vi "Word_Insert_Panel.vi"(0 "Word.Document":refnum<k7>, 1 "Word.InlineShapes":refnum<k7>, 2 "visible area only":bool, 3 "Image depth":u16(ring)=3 items=["B&W", "4 bits", "8 bits", "24 bits"], 5 "VI name":string, 9 "alignment (default)":T1, 11 "Error in":errorcluster, 12 "Insertion point":u16(ring)=1 items=["begining of document", "end of document", "bookmark"], 13 "bookmark name":string, 14 "image file type(.jpg)":enum16{".jpg", ".png"}(ring)) -> (8 "Start out":i32, 10 "End out":i32, 15 "Error out":errorcluster)   [LabVIEW 2020, in "NI_ReportGenerationToolkit.lvlib"]
uses:
  <vilib>/addons/_office/NI_ReportGenerationToolkit.lvlib
  <vilib>/Utility/NIReport.llb/HTML Report Image Alignment.ctl
  <vilib>/Utility/NIReport.llb/NI_ReportGenerationCore.lvlib
panel:
  # "Image"
  # "Position"
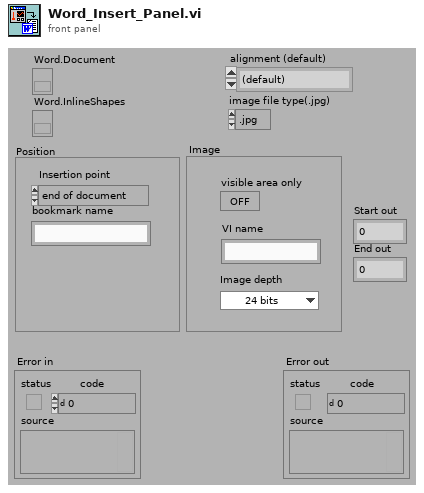
[diagram p1: front panel]
types:
  T1 = typedef "NI_ReportGenerationCore.lvlib/HTML Report Image Alignment.ctl" = enum16{"(default)", "LEFT", "RIGHT", "TOP", "TEXTTOP", "MIDDLE", "ABSMIDDLE", "BASELINE", "BOTTOM", "ABSBOTTOM"}
  T2 = typedef "imagedata.ctl" = cluster{"image type":i32, "image depth":i32, "image":u8[], "mask":u8[], "colors":u32[], "Rectangle":cluster{"left":i16, "top":i16, "right":i16, "bottom":i16}}
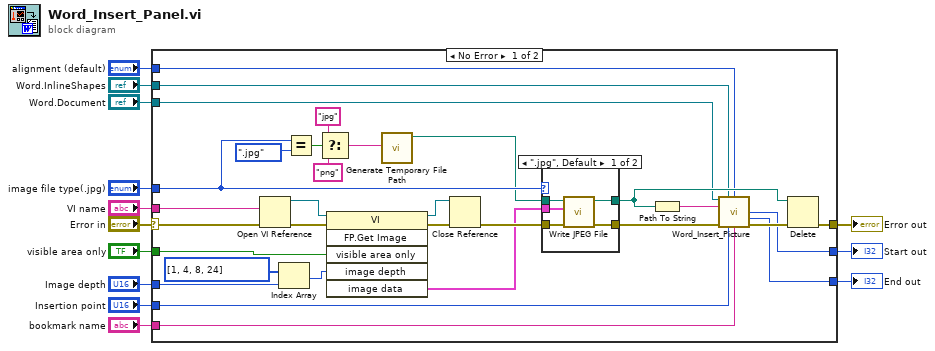
[diagram p0: block diagram]
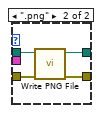
[diagram p2: hidden frame]
diagram:
  n1 = case shown="No Error" "Error in" {
    selector: "Error in" -> [w14 w54]
    tunnel: "VI name" -> [w44 _]
    tunnel: "Image depth" -> [w42 _]
    tunnel: [w41 w54] -> w11
    tunnel: "visible area only" -> [w37 _]
    tunnel: "Word.Document" -> [w35 _]
    tunnel: "Insertion point" -> [w33 _]
    tunnel: "bookmark name" -> [w32 _]
    tunnel: [w29 _] -> w6
    tunnel: [w28 _] -> w5
    tunnel: "alignment (default)" -> [w27 _]
    tunnel: "Word.InlineShapes" -> [w23 _]
    tunnel: "image file type(.jpg)" -> [w17 _]
    frame No Error {
      n2 = Open VI Reference(vi path=w44, error in (no error)=w14) -> (vi reference=w39:refnum<vi>, error out=w36:errorcluster)  [unwired: 4 out]
      n3 = Index Array(array=i32[] [1, 4, 8, 24] ("Array Constant"), index=w42) -> (element=w38:i32)
      n4 = Equal?(x=w17, y=enum16{".jpg", ".png"}.".jpg") -> (x = y?=w21:bool)
      n5 = Select(t="jpg", s=w21, f="png") -> (s? t:f=w20:string)
      n6 = invoke class="VI" method="FP.Get Image"(reference=w39, error in=w36, "visible area only"=w37, "image depth"=w38) -> (reference out=w24:refnum<vi>, error out=w26:errorcluster, "image data"=w15:T2)  [unwired: 2 in, 3 out]
      n7 = call <vilib>:"Generate Temporary File Path.vi"("Temporary File Extension (tmp)"=w20) -> ("Unique Temporary File Path"=w16:path)  [unwired: 1 in, 9 out]
      n8 = Close Reference(reference=w24, error in (no error)=w26) -> (error out=w25:errorcluster)
      n9 = case shown="\".jpg\", Default" w17 {
        tunnel: w16 -> [w47 w53]
        tunnel: w25 -> [w49 w52]
        tunnel: [w48 w51] -> w31
        tunnel: [w46 w50] -> w40
        tunnel: w15 -> [w45 _]
        frame ".jpg", Default {
          n10 = call <vilib>:"Write JPEG File.vi"("error in (no error)"=w49, "image data"=w45, "path to JPEG file"=w47) -> ("error out"=w48:errorcluster, "path"=w46:path)  [unwired: 7 out]
        }
        frame ".png" {
          n11 = call <vilib>:"Write PNG File.vi"("error in (no error)"=w52, "path to PNG file"=w53) -> ("error out"=w51:errorcluster, "path"=w50:path)  [unwired: 1 in, 7 out]
        }
      }
      n12 = Path To String(path=w40) -> (string=w34:string)
      n13 = call <vilib>:"Word_Insert_Picture.vi"("Word.Document"=w35, "Word.InlineShapes"=w23, "alignment (default)"=w27, "Image file path"=w34, "error in (no error)"=w31, "Insertion point"=w33, "bookmark name"=w32) -> ("Start out"=w29:i32, "End out"=w28:i32, "error out 2"=w30:errorcluster)  [unwired: 2 in, 4 out]
      n14 = Delete(path (use dialog)=w40, error in=w30) -> (error out=w41:errorcluster)  [unwired: 5 out]
    }
    frame Error {
    }
  }
  "Error out" <- w11
  "Start out" <- w6
  "End out" <- w5
